vi "Get Function.vi"(0 "VISA resource name":refnum<visa-resource-name>, 11 "error in (no error)":errorcluster) -> (4 "VISA resource name out":refnum<visa-resource-name>, 6 "Function":enum16{"", "3Ø4W", "Parallel", "1Ø3W"}(ring)=enum."3Ø4W", 15 "error out":errorcluster)   [LabVIEW 2016, in "APT 300XAC Series.lvlib"]
doc: "Gets the format of the results to be displayed in the instrument display.\n\n1=3Ø4W\n2=Parallel\n3=1Ø3W"
uses:
  APT 300XAC Series.lvlib
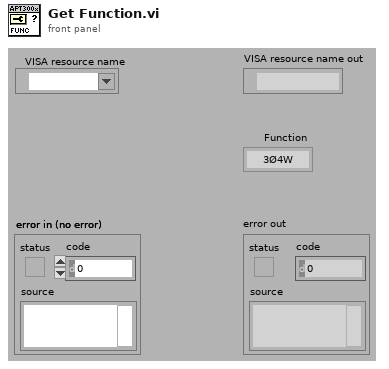
[diagram p1: front panel]
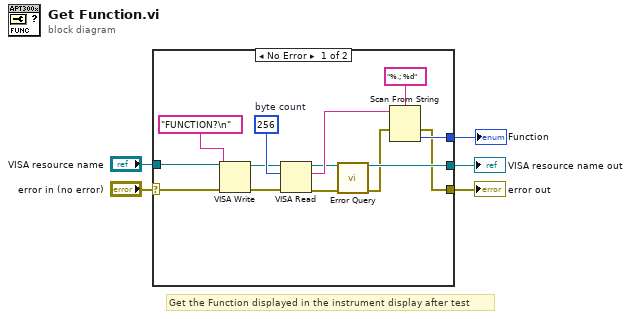
[diagram p0: block diagram]
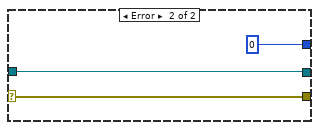
[diagram p2: hidden frame]
diagram:
  # "Get the Function displayed in the instrument display after test"
  n1 = case shown="No Error" "error in (no error)" {
    selector: "error in (no error)" -> [w18 w22]
    tunnel: "VISA resource name" -> [w19 w21]
    tunnel: [w10 w21] -> w4
    tunnel: [w7 w22] -> w3
    tunnel: [w11 0] -> w1
    frame No Error {
      w15 = u32 256  # byte count
      n2 = VISA Write(VISA resource name=w19, write buffer="FUNCTION?\n", error in (no error)=w18) -> (VISA resource name out=w12:refnum<visa-resource-name>, error out=w13:errorcluster)  [unwired: 1 out]
      n3 = VISA Read(VISA resource name=w12, byte count=w15, error in (no error)=w13) -> (VISA resource name out=w9:refnum<visa-resource-name>, read buffer=w14:string, error out=w6:errorcluster)  [unwired: 1 out]
      n4 = call "Error Query.vi"("VISA resource name"=w9, "error in (no error)"=w6) -> ("VISA resource name out"=w10:refnum<visa-resource-name>, "error out"=w8:errorcluster)  [unwired: 10 in, 2 out]
      n5 = Scan From String(format string="%.; %d" ("Format String"), input string=w14, error in=w8) -> (error out=w7:errorcluster, output 1=w11:i32)  [unwired: 2 in, 2 out]
    }
    frame Error {
    }
  }
  "error out" <- w3
  "VISA resource name out" <- w4
  "Function" <- w1
